vi "Release.vi"(8 "error in (no error)":errorcluster, 11 "YP03-60_X in":refnum<class "YP03-60_X.lvclass">) -> (0 "error out":errorcluster)   [LabVIEW 2020, in "PowerControl.lvlib" / "YP03-60_X.lvclass"]
uses:
  YP03-60_X.lvclass
  YP03-60_X.lvclass/YP03-60_X.ctl
  VirtualPower/VirtualPower.lvclass
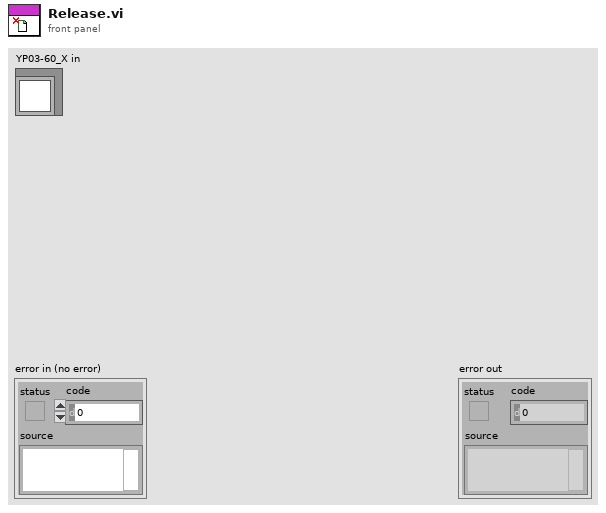
[diagram p1: front panel]
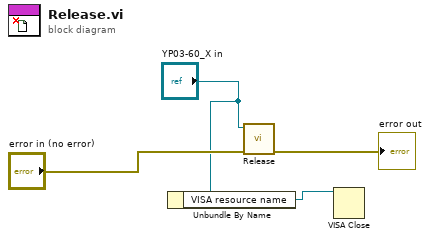
[diagram p0: block diagram]
diagram:
  n1 = Unbundle By Name("YP03-60_X in") -> ("VISA resource name"=w1:refnum<visa-resource-name>)
  n2 = call-parent "Release.vi"("error in (no error)"="error in (no error)", "VirtualPower in"="YP03-60_X in") -> ("error out"=→"error out":errorcluster)  [unwired: 9 in]
  n3 = VISA Close(VISA resource name=w1) -> ()  [unwired: 1 in, 1 out]
